vi "Motion_Wait for Gantry Home.vi"(8 "error in":errorcluster, 10 "timeout (60s)":dbl[unit]=60.0 caption="Time Target (s)" format="%.1f", 11 "TCP refnum":refnum<k5>) -> (0 "error out":errorcluster, 1 "Gantry At Home":bool, 2 "elapsed time":dbl[unit]=nan format="%.1f", 3 "TCP refnum dup":refnum<k5>, 4 "timeout error":bool, 5 "done":bool)   [LabVIEW 2010]
panel:
  in  "poll interval (0.1s)":dbl[unit]=0.1
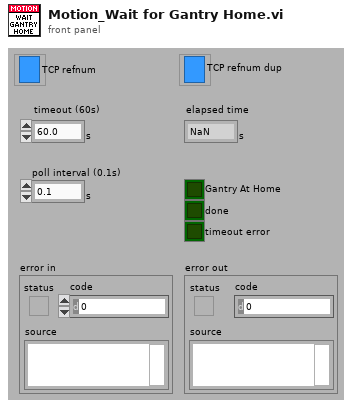
[diagram p1: front panel]
types:
  T1 = cluster{"Gantry Enabled":bool, "Gantry Power Error":bool, "Gantry Moving":bool, "Gantry At Position":bool, "Gantry Goto Error":bool, "Gantry Goto Aborted":bool, "Gantry Homing":bool, "Gantry Home Error":bool, "Gantry Home Required":bool, "Gantry Home Aborted":bool, "Gantry General Alarm":bool, "Motion Alarm":bool}
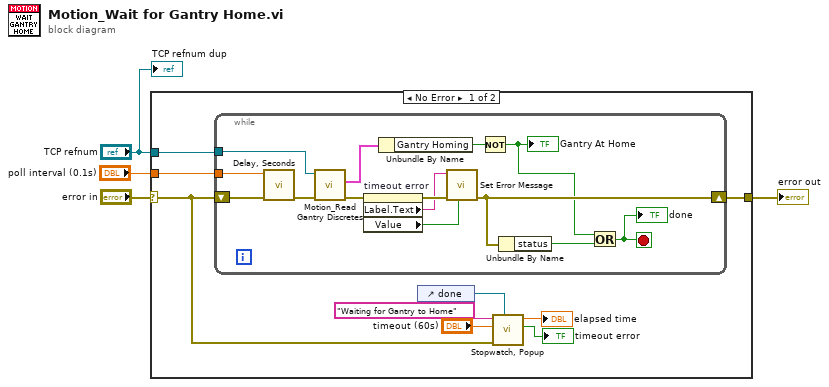
[diagram p0: block diagram]
diagram:
  n1 = case shown="No Error" "error in" {
    selector: "error in" -> [w6 w28]
    tunnel: "TCP refnum" -> [w8 _]
    tunnel: [w7 w28] -> w4
    tunnel: "poll interval (0.1s)" -> [w5 _]
    frame No Error {
      n2 = while {
        tunnel: w8 -> [w27]
        shift-right: [w19] -> w7
        shift-left: w6 -> [w25]
        tunnel: w5 -> [w17]
        stop <- w14 stop-if-true
        n3 = call "Delay, Seconds.vi"("error in"=w25, "delay"=w17) -> ("error out"=w24:errorcluster)  [unwired: 5 in, 1 out]
        n4 = call "Motion_Read Gantry Discretes.vi"("error in (no error)"=w24, "TCP Connection Refnum in"=w27) -> ("error out"=w23:errorcluster, "Gantry Discretes"=w26:T1)  [unwired: 7 in, 1 out]
        n5 = property on="timeout error" class="Bool (strict)"(error in=w23) -> (error out=w22:errorcluster, "Label.Text"=w20:string, "Value"=w21:bool)  [unwired: 1 in, 1 out]
        n6 = Unbundle By Name(w26) -> ("Gantry Homing"=w16:bool)
        n7 = call "Set Error Message.vi"("enable (T)"=w21, "error in"=w22, "message"=w20) -> ("error out"=w19:errorcluster)  [unwired: 5 in]
        n8 = Not(x=w16) -> (.not. x?=w15:bool)
        "Gantry At Home" <- w15
        n9 = Unbundle By Name(w19) -> ("status"=w18:bool)
        n10 = Or(x=w15, y=w18) -> (x .or. y?=w14:bool)
        "done" <- w14
      }
      n11 = control-ref of="done"() -> (w12:refnum<vi>)
      n12 = call "Stopwatch, Popup.vi"("Stop (Bool) Refnum"=w12, "error in (no error)"=w6, "Time Target"="timeout (60s)", "Front Panel Window:Title"="Waiting for Gantry to Home") -> ("Time has Elapsed"=→"timeout error":bool, "Elapsed Time (Knob)"=→"elapsed time":dbl[unit])  [unwired: 5 in, 1 out]
    }
    frame Error {
    }
  }
  "error out" <- w4
  "TCP refnum dup" <- "TCP refnum"
